vi "TF - Transfer Function and Coherence.vi"(0 "reference in":refnum<class "GSwFormDSP.lvclass">, 5 "error in (no error)":errorcluster) -> (14 "reference out":refnum<class "GSwFormDSP.lvclass">, 19 "error out":errorcluster)   [LabVIEW 2020, in "GSwFormDSP.lvclass"]
uses:
  GSwFormDSP.lvclass
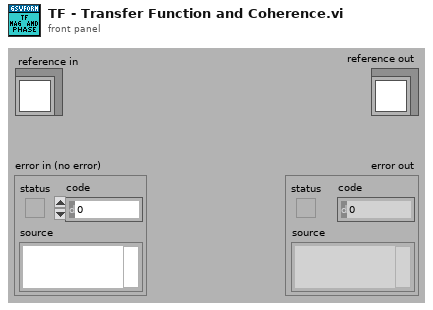
[diagram p1: front panel]
types:
  T1 = typedef "GSwFormDSP.lvclass/ObjectAttributesRef.ctl" = refnum<data-value>
  T2 = typedef "GSwFormDSP.lvclass/ObjectAttributes.ctl" = cluster{"Wform Ref":refnum<data-value>, "Nb Signals":i32, "Spectral Function Parameters":T3, "FFT":waveform(cdb)[], "Nb FFT":i32, "Nb Averages":i32[], "Reference Indexes":i32[], "Response Indexes":i32[], "Coherence":waveform(dbl)[], "TDF Parameters":T5, "DAQ":cluster{"Duration (sec)":dbl, "Buffer Size (Samples)":i32, "Offset (Samples)":i32}, "Filter Impulse Response (TDF)":waveform(dbl), "Sound Playback":T6}
  T3 = typedef "GSwFormDSP.lvclass/Spectral Parameters.ctl" = cluster{"Frequency resolution (Hz)":dbl, "Overlap":dbl, "Window":T4}
  T4 = typedef "NI_AALPro.lvlib/windowTd.ctl" = u32
  T5 = typedef "GSwFormDSP.lvclass/TDF Parameters.ctl" = cluster{"Filter":enum32{"Lowpass", "Highpass", "Bandpass", "Bandstop"}, "Type:":enum16{"Butterworth", "Chebyshev", "Inv Chebyshev", "Elliptic", "Bessel"}, "LP cutoff freq":dbl, "HP cutoff freq":dbl, "Order":i32, "passband ripple (dB)":dbl, "stopband attenuation (dB)":dbl, "Phaseless Filter":bool, "Include Fade IN and OUT":bool}
  T6 = typedef "GSwFormDSP.lvclass/Sound Playback.ctl" = cluster{"Timer start (ms)":u32, "task ID":T7, "Cursor Init Location (s)":dbl, "SC Volume":dbl}
  T7 = typedef "Sound Output Task ID.ctl" = u32
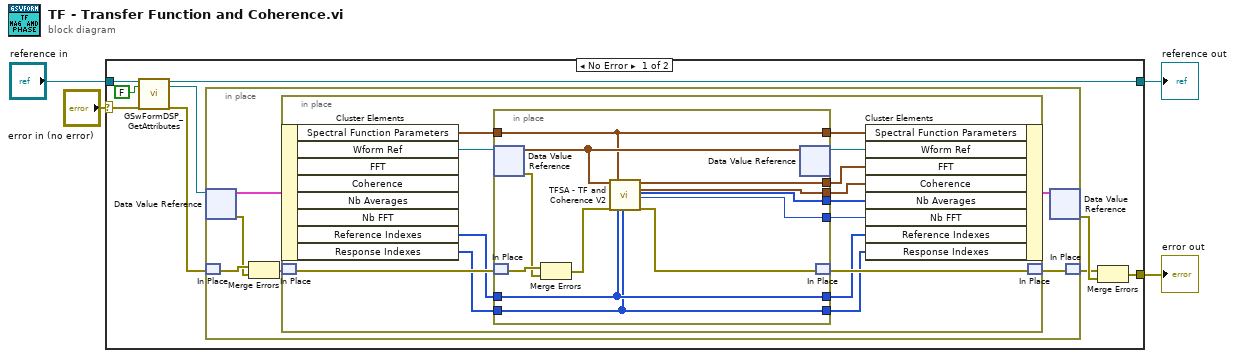
[diagram p0: block diagram]
diagram:
  n1 = case shown="No Error" "error in (no error)" {
    selector: "error in (no error)" -> [w10 w47]
    tunnel: [w13 w47] -> w3
    tunnel: [w11 w46] -> w1
    tunnel: "reference in" -> [w12 w46]
    frame No Error {
      n2 = call "GSwFormDSP_GetAttributes.vi"("reference in"=w12, "return data? (T)"=FALSE, "error in (no error)"=w10) -> ("reference out"=w11:refnum<class "GSwFormDSP.lvclass">, "attributes ref"=w8:T1, "error out"=w7:errorcluster)  [unwired: 13 in, 1 out]
      n3 = in-place {
        n4 = in-place-dvr #1(w8) -> (w18:T2, w16:errorcluster)
        n5 = in-place-match #2(w7) -> (w17:errorcluster)
        n6 = Merge Errors(w17, w16) -> (w15:errorcluster)
        n7 = in-place {
          n8 = in-place-cluster #3(w18) -> ("Spectral Function Parameters"=w23:T3, "Wform Ref"=w33:refnum<data-value>, "Reference Indexes"=w27:i32[], "Response Indexes"=w24:i32[])  [unwired: 4 out]
          n9 = in-place-match #4(w15) -> (w31:errorcluster)
          n10 = in-place {
            in-place-border: w27 -> [w38]
            in-place-border: [w38] -> w26
            in-place-border: [w40] -> w29
            in-place-border: [w39] -> w28
            in-place-border: [w37] -> w25
            in-place-border: w24 -> [w37]
            in-place-border: w23 -> [w36]
            in-place-border: [w36] -> w22
            in-place-border: [w35] -> w21
            in-place-border: [w34] -> w20
            n11 = in-place-dvr #5(w33) -> (w41:waveform(dbl)[], w44:errorcluster)
            n12 = in-place-match #6(w31) -> (w45:errorcluster)
            n13 = Merge Errors(w45, w44) -> (w43:errorcluster)
            n14 = call "TFSA - TF and Coherence V2.vi"("wForms IN"=w41, "error in (no error)"=w43, "Spectral Function Parameters"=w36, "Reference Indexes"=w38, "Response Indexes"=w37) -> ("TF OUT"=w40:waveform(cdb)[], "Coherence"=w39:waveform(dbl)[], "Nb Averages"=w35:i32[], "Nb TF"=w34:i32, "error out"=w42:errorcluster)  [unwired: 10 in]
            n15 = in-place-dvr #5(w41) -> (w32:refnum<data-value>)  [unwired: 1 out]
            n16 = in-place-match #6(w42) -> (w30:errorcluster)
          }
          n17 = in-place-cluster #3("Spectral Function Parameters"=w22, "Wform Ref"=w32, "FFT"=w29, "Coherence"=w28, "Nb Averages"=w21, "Nb FFT"=w20, "Reference Indexes"=w26, "Response Indexes"=w25) -> (w19:T2)
          n18 = in-place-match #4(w30) -> (w14:errorcluster)
        }
        n19 = in-place-dvr #1(w19) -> (w9:errorcluster)  [unwired: 1 out]
        n20 = in-place-match #2(w14) -> (w6:errorcluster)
      }
      n21 = Merge Errors(w6, w9) -> (w13:errorcluster)
    }
    frame Error {
    }
  }
  "error out" <- w3
  "reference out" <- w1
